vi "Generate JSON Schema VCluster.vi"(6 "strict?":bool, 8 "error in (no error)":errorcluster, 11 "type":variant) -> (0 "error out":errorcluster, 3 "json schema cluster":variant)   [LabVIEW 2020]
uses:
  <vilib>/Utility/Data Type/NI_Data Type.lvlib
  <userlib>/_OpenG.lib/lvdata/lvdata.llb/openg_variant.lvlib
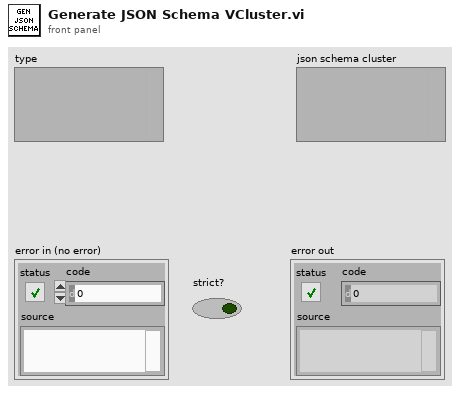
[diagram p1: front panel]
types:
  T1 = typedef "NI_Data Type.lvlib/Data Type.ctl" = enum8{"Invalid Type", "Void", "I8", "I16", "I32", "I64", "U8", "U16", "U32", "U64", "Single Float", "Double Float", "Extended Float", "Single Complex", "Double Complex", "Extended Complex", "Enum U8", "Enum U16", "Enum U32", "Enum U64", "Single Float With Unit", "Double Float With Unit", "Extended Float With Unit", "Single Complex with Unit", "Double Complex with Unit", "Extended Complex with Unit", "Boolean", "String", "Path", "Picture", "Tag", "Array", "Cluster", "Variant", "LV Variant", "Waveform", "Timestamp", "Digital Waveform", "Digital Data", "ExpressData", "Refnum", "External Data", "VI", "Poly VI", "LabVIEW Class Instance", "Fixed Point", "Set Collection", "Map Collection"}
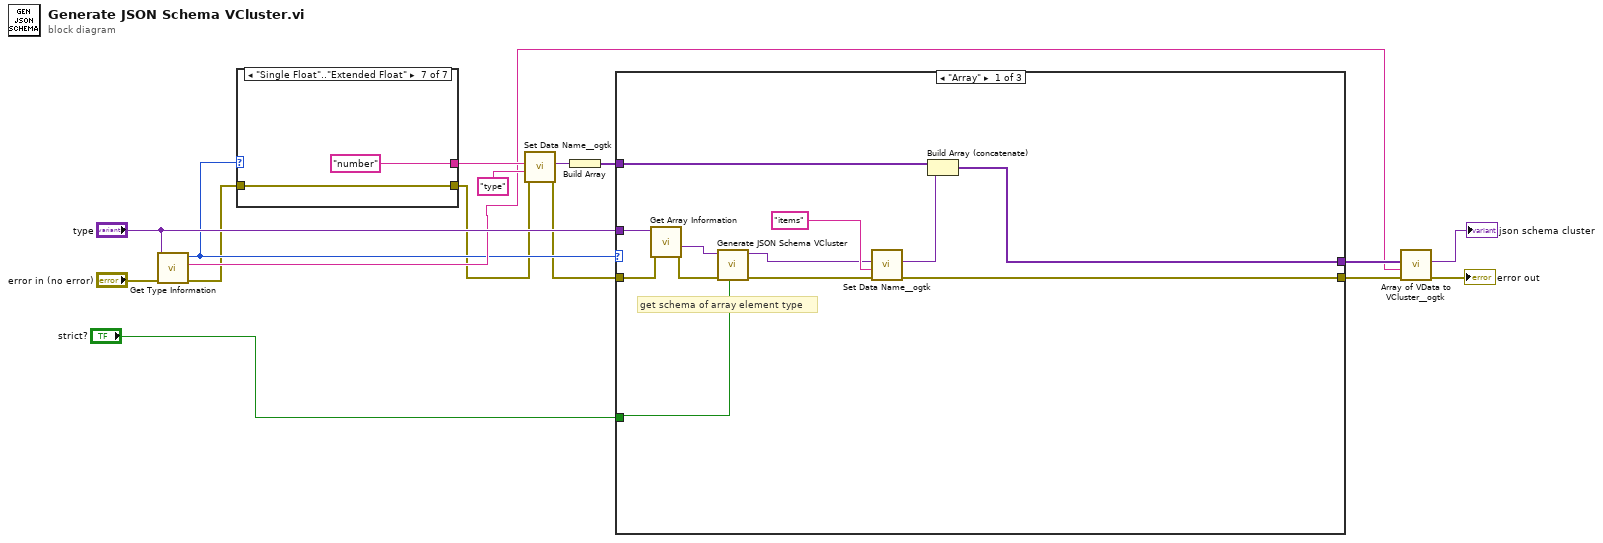
[diagram p0: block diagram]
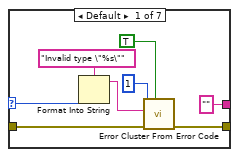
[diagram p2: hidden frame]
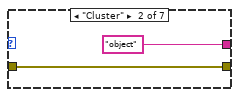
[diagram p3: hidden frame]
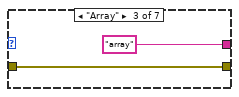
[diagram p4: hidden frame]
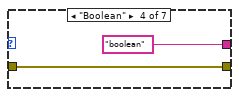
[diagram p5: hidden frame]
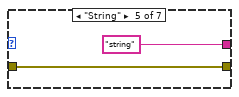
[diagram p6: hidden frame]
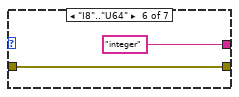
[diagram p7: hidden frame]
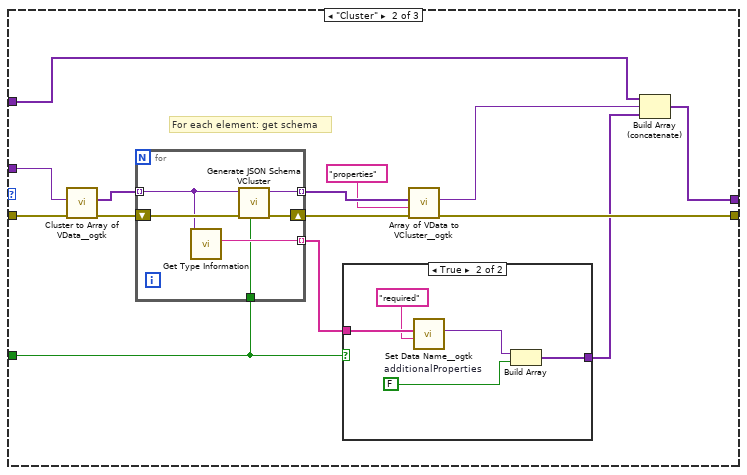
[diagram p8: hidden frame]
diagram:
  n1 = call <vilib>:"Get Type Information.vi"("error in (no error)"="error in (no error)", "variant"="type") -> ("error out"=w6:errorcluster, "name"=w8:string, "type"=w7:T1)  [unwired: 5 in, 2 out]
  n2 = case shown="\"Single Float\"..\"Extended Float\"" w7 {
    selector: w7 -> [w20 _ _ _ _ _ _]
    tunnel: ["" ("name") "object" ("name") "array" ("name") "boolean" ("name") "string" ("name") "integer" ("name") "number" ("name")] -> w14
    tunnel: [w22 w25 w27 w29 w31 w33 w35] -> w4
    tunnel: w6 -> [w24 w25 w27 w29 w31 w33 w35]
    frame Default {
      n3 = Format Into String(format string="Invalid type \"%s\"", w20) -> (resulting string=w18:string)  [unwired: 2 in, 1 out]
      n4 = call <vilib>:"Error Cluster From Error Code.vi"("show call chain? (False)"=TRUE, "error in (no error)"=w24, "error message (\"\")"=w18, "error code (0)"=1) -> ("error out"=w22:errorcluster)  [unwired: 5 in]
    }
    frame "Cluster" {
    }
    frame "Array" {
    }
    frame "Boolean" {
    }
    frame "String" {
    }
    frame "I8".."U64" {
    }
    frame "Single Float".."Extended Float" {
    }
  }
  n5 = call <userlib>:"Set Data Name__ogtk.vi"("error in (no error)"=w4, "Data Name"="type" ("name"), "Data"=w14) -> ("error out"=w3:errorcluster, "Renamed Data"=w12:variant)  [unwired: 7 in]
  n6 = Build Array(w12) -> (w11:variant[])
  n7 = case shown="\"Array\"" w7 {
    tunnel: [w42 w56 w75] -> w10
    tunnel: "type" -> [w48 w62 _]
    tunnel: w11 -> [w43 w60 w75]
    tunnel: w3 -> [w41 w55 w74]
    tunnel: [w38 w52 w74] -> w2
    tunnel: "strict?" -> [w37 w49 _]
    frame "Array" {
      # "get schema of array element type"
      n8 = call <vilib>:"Get Array Information.vi"("error in (no error)"=w41, "variant"=w48) -> ("error out"=w40:errorcluster, "array element data type"=w47:variant)  [unwired: 6 in, 2 out]
      n9 = call "Generate JSON Schema VCluster.vi"("strict?"=w37, "error in (no error)"=w40, "type"=w47) -> ("error out"=w39:errorcluster, "json schema cluster"=w45:variant)  [unwired: 7 in]
      n10 = call <userlib>:"Set Data Name__ogtk.vi"("error in (no error)"=w39, "Data Name"="items" ("name"), "Data"=w45) -> ("error out"=w38:errorcluster, "Renamed Data"=w44:variant)  [unwired: 7 in]
      n11 = Build Array (concatenate)(w43, w44) -> (w42:variant[])
    }
    frame "Cluster" {
      # "For each element: get schema"
      n12 = call <userlib>:"Cluster to Array of VData__ogtk.vi"("error in (no error)"=w55, "Cluster"=w62) -> ("error out"=w54:errorcluster, "Array of VData"=w61:variant[])  [unwired: 8 in]
      n13 = for {
        tunnel: w61 -> [w70] mode=indexing
        tunnel: [w73] -> w59 mode=indexing
        shift-right: [w71] -> w53
        shift-left: w54 -> [w72]
        tunnel: [w69] -> w51 mode=indexing
        tunnel: w49 -> [w68]
        n14 = call <vilib>:"Get Type Information.vi"("variant"=w70) -> ("name"=w69:string)  [unwired: 6 in, 4 out]
        n15 = call "Generate JSON Schema VCluster.vi"("strict?"=w68, "error in (no error)"=w72, "type"=w70) -> ("error out"=w71:errorcluster, "json schema cluster"=w73:variant)  [unwired: 7 in]
      }
      n16 = case shown="True" w49 {
        tunnel: w51 -> [_ w67]
        tunnel: [_ w63] -> w50
        frame False {
        }
        frame True {
          w64 = FALSE  # additionalProperties
          n17 = call <userlib>:"Set Data Name__ogtk.vi"("Data Name"="required" ("name"), "Data"=w67) -> ("Renamed Data"=w65:variant)  [unwired: 8 in, 1 out]
          n18 = Build Array(w65, w64) -> (w63:variant[])
        }
      }
      n19 = call <userlib>:"Array of VData to VCluster__ogtk.vi"("error in (no error)"=w53, "Cluster Name"="properties" ("name"), "Array"=w59) -> ("error out"=w52:errorcluster, "VCluster"=w57:variant)  [unwired: 7 in]
      n20 = Build Array (concatenate)(w60, w57, w50) -> (w56:variant[])
    }
    frame Default {
    }
  }
  n21 = call <userlib>:"Array of VData to VCluster__ogtk.vi"("error in (no error)"=w2, "Cluster Name"=w8, "Array"=w10) -> ("error out"=→"error out":errorcluster, "VCluster"=→"json schema cluster":variant)  [unwired: 7 in]
